vi "Write Roles.vi"(8 "error in (no error)":errorcluster, 10 "Roles":T1, 11 "TimeoutPlay in":refnum<class "TimeoutPlay.lvclass">) -> (0 "error out":errorcluster, 3 "TimeoutPlay out":refnum<class "TimeoutPlay.lvclass">)   [LabVIEW 2020, in "TimeoutPlay.lvclass"]
uses:
  TimeoutPlay.lvclass
  TimeoutRole_class/TimeoutRole.lvclass
  TimeoutPlay.lvclass/TimeoutPlay.ctl
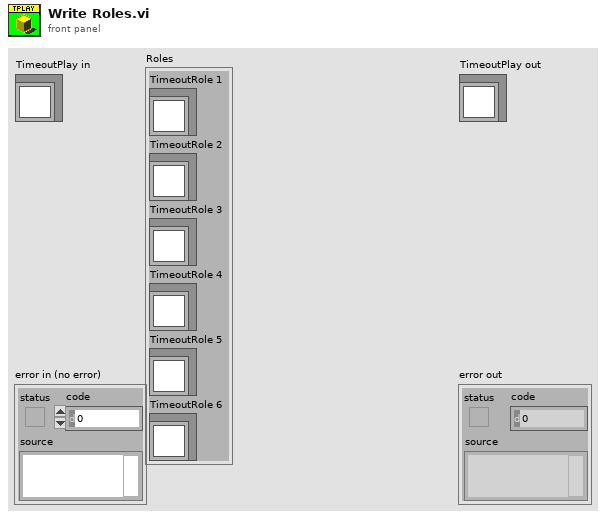
[diagram p1: front panel]
types:
  T1 = cluster{"TimeoutRole 1":refnum<class "TimeoutRole.lvclass">, "TimeoutRole 2":refnum<class "TimeoutRole.lvclass">, "TimeoutRole 3":refnum<class "TimeoutRole.lvclass">, "TimeoutRole 4":refnum<class "TimeoutRole.lvclass">, "TimeoutRole 5":refnum<class "TimeoutRole.lvclass">, "TimeoutRole 6":refnum<class "TimeoutRole.lvclass">}
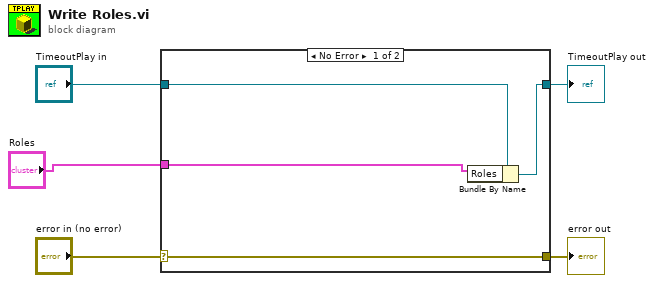
[diagram p0: block diagram]
diagram:
  n1 = case shown="No Error" "error in (no error)" {
    selector: "error in (no error)" -> [w9 w10]
    tunnel: [w9 w10] -> w4
    tunnel: [w7 w11] -> w2
    tunnel: "TimeoutPlay in" -> [w8 w11]
    tunnel: "Roles" -> [w6 _]
    frame No Error {
      n2 = Bundle By Name(cluster=w8, "Roles"=w6) -> (w7:refnum<class "TimeoutPlay.lvclass">)
    }
    frame Error {
    }
  }
  "error out" <- w4
  "TimeoutPlay out" <- w2
